vi "ALLOutput set.vi"(7 "ALLOutput":bool, 8 "error in (no error)":errorcluster, 9 "VISA resource name":refnum<visa-resource-name>) -> (0 "error out":errorcluster, 1 "VISA resource name out":refnum<visa-resource-name>)   [LabVIEW 2012, in "GPP.lvlib"]
uses:
  GPP.lvlib
  Function/VISA_COMMON.ctl
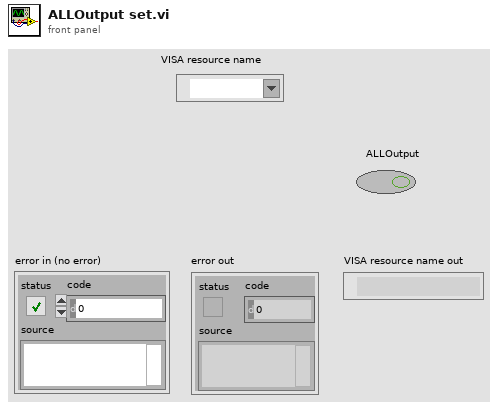
[diagram p1: front panel]
types:
  T1 = typedef "GPP.lvlib/VISA_COMMON.ctl" = enum16{"Initial", "Write CMD", "Read Result", "Read History", "Close"}
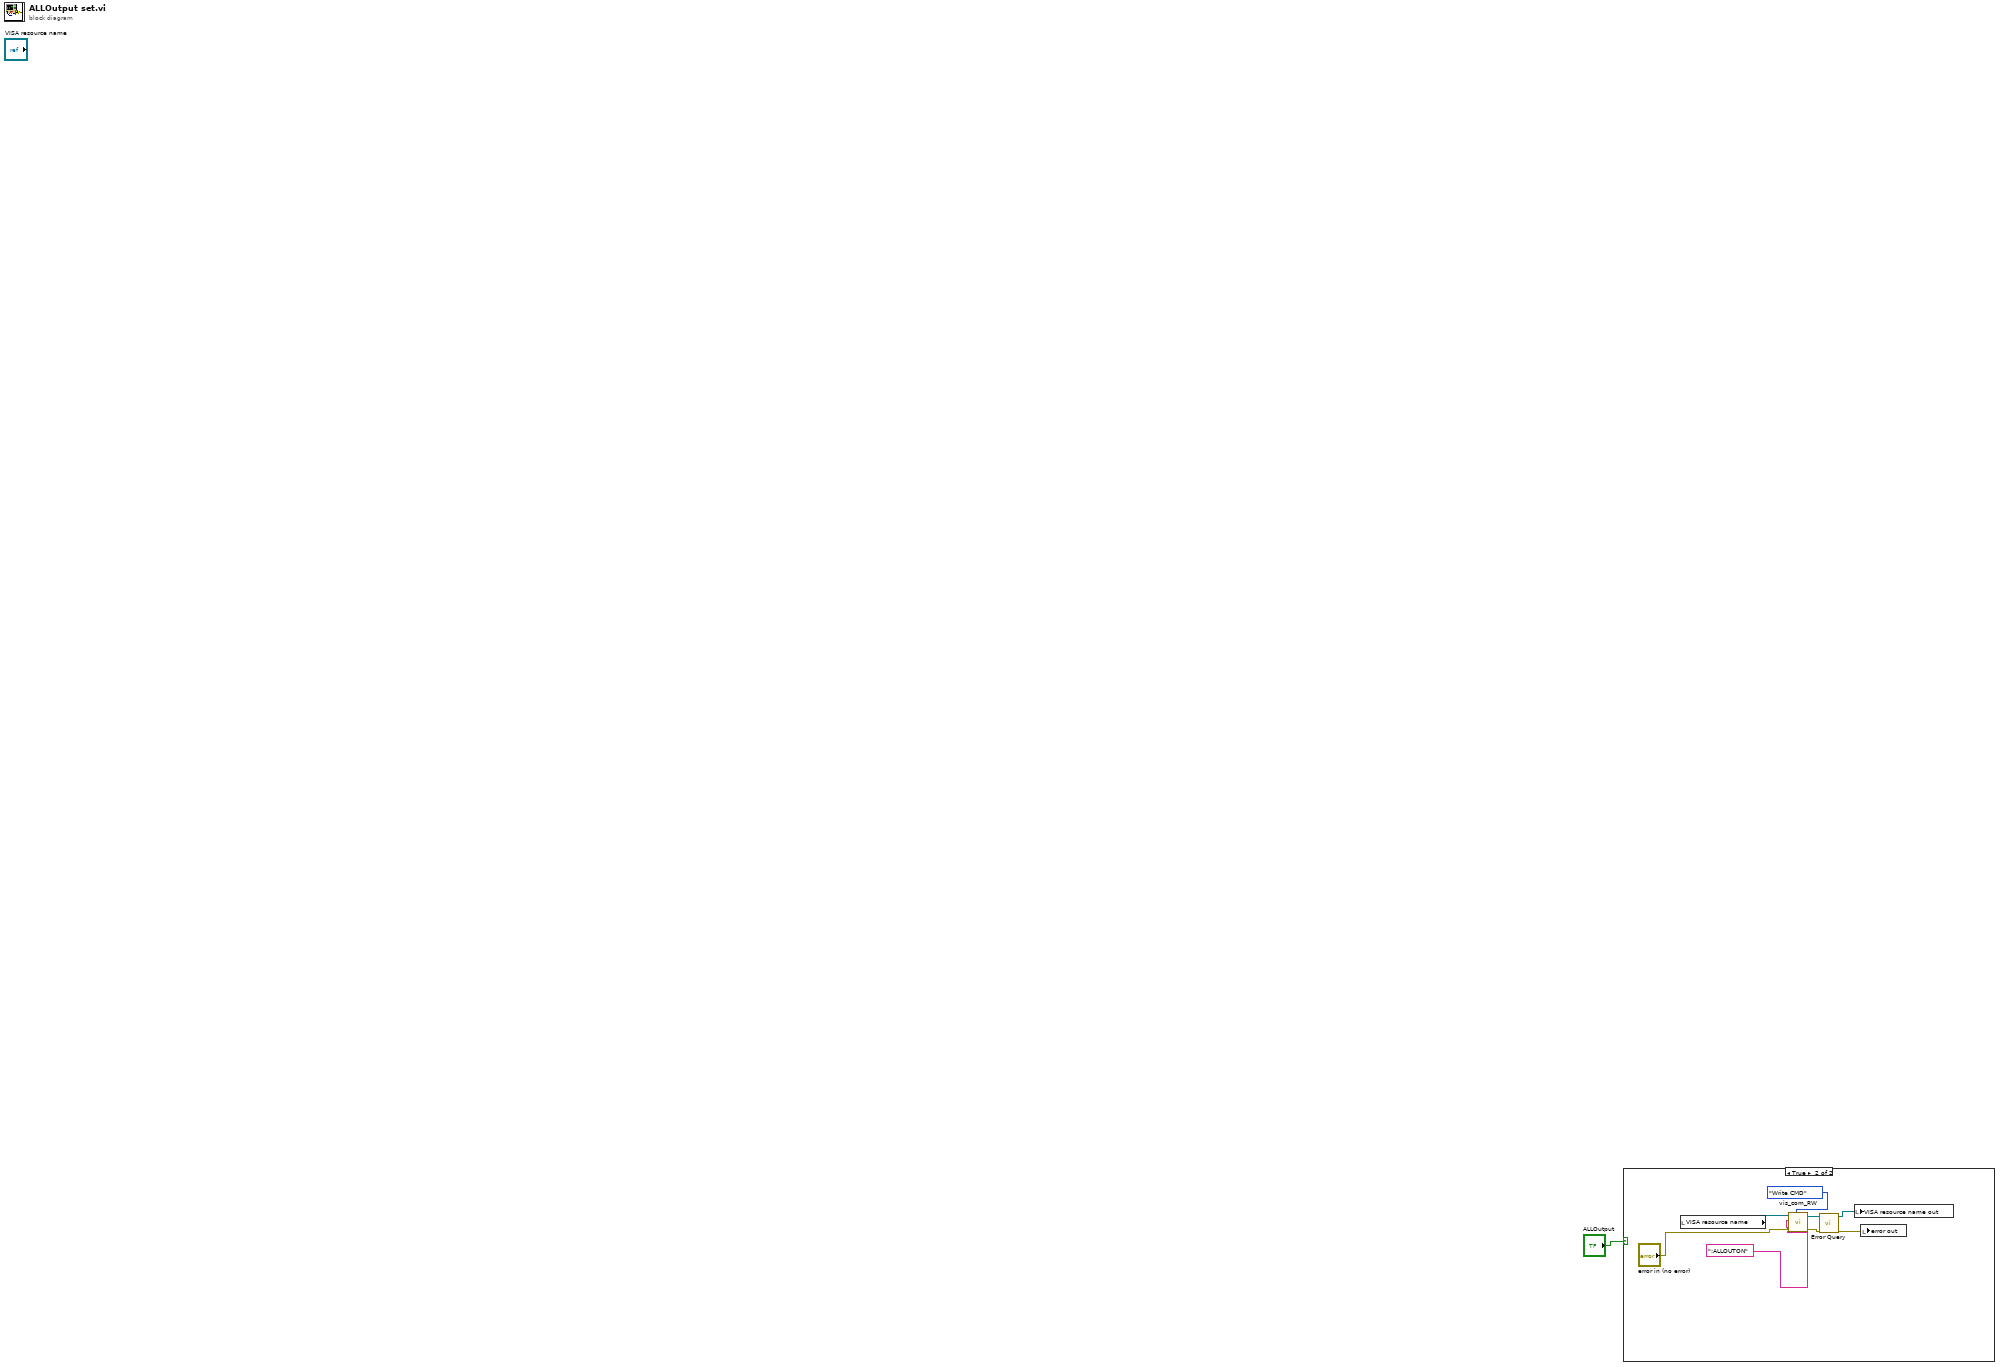
[diagram p0: block diagram]
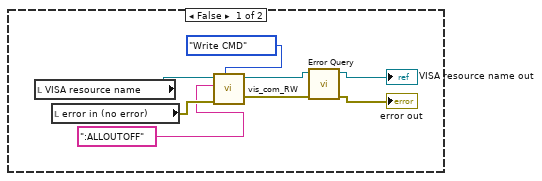
[diagram p2: hidden frame]
diagram:
  n1 = case shown="True" "ALLOutput" {
    frame False {
      n2 = local read "VISA resource name"() -> (w9:refnum<visa-resource-name>)
      n3 = local read "error in (no error)"() -> (w8:errorcluster)
      n4 = call "vis_com_RW.vi"("Funciton"=VISA_COMMON."Write CMD", "error in (no error)"=w8, "CMD String"=":ALLOUTOFF", "VISA resource in"=w9) -> ("error out"=w4:errorcluster, "VISA resource out"=w5:refnum<visa-resource-name>)  [unwired: 5 in, 1 out]
      n5 = call "Error Query.vi"("error in (no error)"=w4, "VISA resource name"=w5) -> ("error out"=→"error out":errorcluster, "VISA resource name out"=→"VISA resource name out":refnum<visa-resource-name>)  [unwired: 6 in, 2 out]
    }
    frame True {
      n6 = local read "VISA resource name"() -> (w17:refnum<visa-resource-name>)
      n7 = call "vis_com_RW.vi"("Funciton"=VISA_COMMON."Write CMD", "error in (no error)"="error in (no error)", "CMD String"=":ALLOUTON", "VISA resource in"=w17) -> ("error out"=w13:errorcluster, "VISA resource out"=w12:refnum<visa-resource-name>)  [unwired: 5 in, 1 out]
      n8 = call "Error Query.vi"("error in (no error)"=w13, "VISA resource name"=w12) -> ("error out"=w14:errorcluster, "VISA resource name out"=w15:refnum<visa-resource-name>)  [unwired: 6 in, 2 out]
      n9 = local write "VISA resource name out"(w15) -> ()
      n10 = local write "error out"(w14) -> ()
    }
  }
